vi "sub-level-1.vi"() -> ()   [LabVIEW 2017]
panel:
  out "String":string
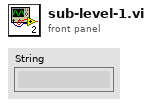
[diagram p1: front panel]
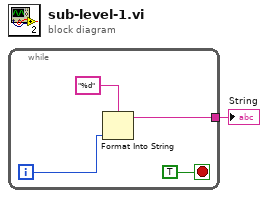
[diagram p0: block diagram]
diagram:
  n1 = while {
    tunnel: [w2] -> w1
    i -> [w4]
    stop <- TRUE stop-if-true
    n2 = Format Into String(format string="%d", w4) -> (resulting string=w2:string)  [unwired: 2 in, 1 out]
  }
  "String" <- w1
